vi "GenCylinder.vi"(11 "Solid Horizon Path.PNG":path=path "C:/Users/uksayerr/Documents/My LabView/Content Creation/artificial horizon/FixedHorizonTrans.png") -> (3 "SceneObject out":refnum<vi>)   [LabVIEW 2010]
uses:
  <vilib>/picture/3D Picture Control/NI_3D Picture Control.lvlib
panel:
  # "Generates the rotating drum with the picture \nat the path specified below"
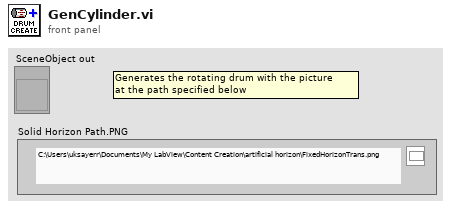
[diagram p1: front panel]
types:
  T1 = enum16{"Inherit Value", "No Culling", "Cull Back Face", "Cull Front Face", "Cull Both Faces"}
  T2 = enum16{"No Filtration", "Linear Filtration", "Simple Mipmap Filtration", "Bilinear Filtration", "Trilinear Filtration"}
  T3 = enum16{"As a Decal", "With Modulation", "With Blending", "As a replacement"}
  T4 = typedef "imagedata.ctl" = cluster{"image type":i32, "image depth":i32, "image":u8[], "mask":u8[], "colors":u32[], "Rectangle":cluster{"left":i16, "top":i16, "right":i16, "bottom":i16}}
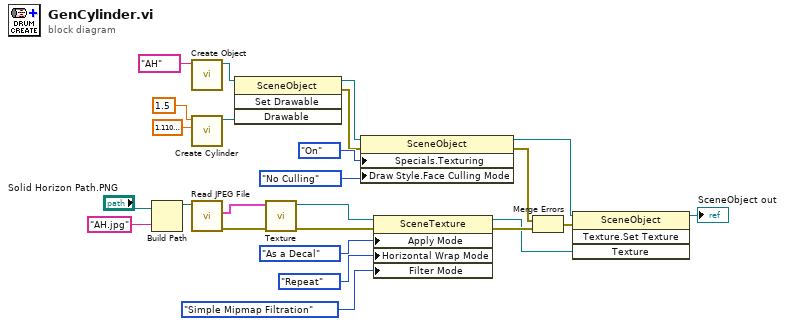
[diagram p0: block diagram]
diagram:
  n1 = Build Path(base path="Solid Horizon Path.PNG", name or relative path="AH.jpg") -> (appended path=w1:path)
  n2 = call <vilib>:"Create Object.vi"("Name"="AH") -> ("Scene:New Object"=w14:refnum<vi>)  [unwired: 1 in, 9 out]
  n3 = call <vilib>:"Create Cylinder.vi"("Radius"=sgl 1.11 ("Detail"), "Height"=sgl 1.5 ("Radius")) -> ("New Cylinder Refnum"=w10:refnum<vi>)  [unwired: 8 in, 1 out]
  n4 = call <vilib>:"Read JPEG File.vi"("path to JPEG file"=w1) -> ("error out"=w4:errorcluster, "image data"=w5:T4)  [unwired: 8 in, 1 out]
  n5 = invoke class="SceneObject" method="Set Drawable"(reference=w14, "Drawable"=w10) -> (reference out=w11:refnum<vi>, error out=w12:errorcluster)  [unwired: 2 in, 2 out]
  n6 = call <vilib>:"Texture.vi"("error in (no error)"=w4, "Image"=w5) -> ("error out"=w22:errorcluster, "New Texture Refnum"=w15:refnum<vi>)  [unwired: 8 in]
  n7 = property class="SceneObject"(reference=w11, error in=w12, "Specials.Texturing"=enum16{"Inherit Value", "Off", "On"}."On" ("Specials:Texturing"), "Draw Style.Face Culling Mode"=T1."No Culling" ("Draw Style:Face Culling Mode")) -> (reference out=w19:refnum<vi>, error out=w23:errorcluster)
  n8 = property class="SceneTexture"(reference=w15, error in=w22, "Apply Mode"=T3."As a Decal", "Horizontal Wrap Mode"=enum16{"Clamp", "Repeat"}."Repeat", "Filter Mode"=T2."Simple Mipmap Filtration") -> (reference out=w20:refnum<vi>, error out=w24:errorcluster)
  n9 = Merge Errors(w23, w24) -> (w21:errorcluster)
  n10 = invoke class="SceneObject" method="Texture.Set Texture"(reference=w19, error in=w21, "Texture"=w20) -> (reference out=→"SceneObject out":refnum<vi>)  [unwired: 1 in, 3 out]
